vi "HTML Hierarhy Close Branch.vi"(8 "error in":errorcluster) -> (0 "error out":errorcluster)   [LabVIEW 2014, in "lvprj2html.lvlib"]
uses:
  lvprj2html.lvlib
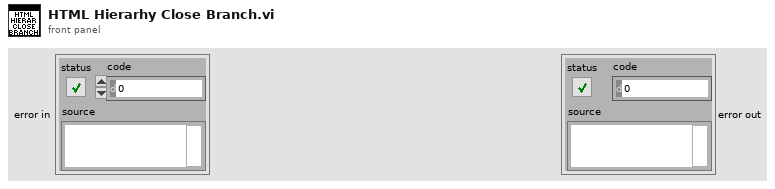
[diagram p1: front panel]
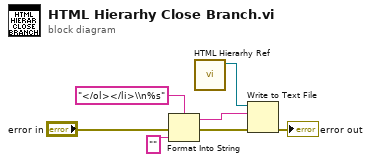
[diagram p0: block diagram]
diagram:
  n1 = Format Into String(format string="</ol></li>\\n%s" ("text"), error in="error in", "" ("input 1")) -> (resulting string=w5:string, error out=w2:errorcluster)  [unwired: 1 in]
  n2 = call "HTML Hierarhy Ref.vi"() -> ("Byte Stream File out"=w7:refnum<file>)  [unwired: 11 in]
  n3 = Write to Text File(file (use dialog)=w7, text=w5, error in=w2) -> (error out=→"error out":errorcluster)  [unwired: 1 in, 2 out]
